vi "CRYRef nums global.vi"() -> ()   [LabVIEW 2013]
panel:
  out "CRY6181 One VI ref":refnum<vi>
  out "AddStep VI ref":refnum<vi>
  out "Run project VI ref":refnum<vi>
  out "Post Sub VI ref":refnum<vi>
  out "Stimulus Sub VI ref":refnum<vi>
  in  "vi reference":refnum<vi>
  out "Step Edit VI ref nums":refnum<vi>[](array[refnum])
  in  "LVserial init ports":i32[](array[numeric]) min=1 max=99
  in  "VISA serial ports":T1(array[cluster]) {"COM port (1 = COM1, etc.)" min=1 max=99}
  in  "DIO VI ref nums":T2
  in  "DIO task IDs":u32[](array[numeric])
  out "Step Run VI ref nums":refnum<vi>[](array[refnum])
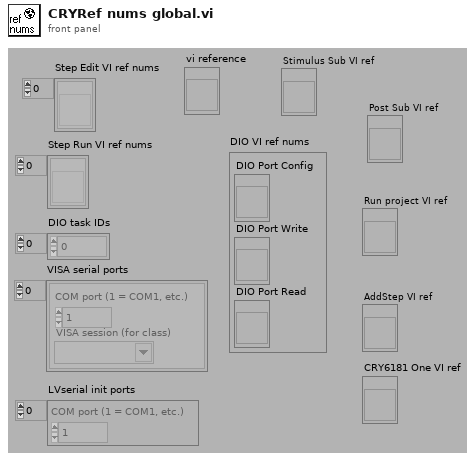
[diagram p1: front panel]
types:
  T1 = cluster{"COM port (1 = COM1, etc.)":i32, "VISA session (for class)":refnum<visa-resource-name>}[]
  T2 = cluster{"DIO Port Config":refnum<vi>, "DIO Port Write":refnum<vi>, "DIO Port Read":refnum<vi>}
diagram:
